vi "Pool.Destroy FIFO.vi"(8 "error in (no error)":errorcluster, 11 "Pool in":refnum<class "Pool.lvclass">) -> (0 "error out":errorcluster, 3 "Pool out":refnum<class "Pool.lvclass">)   [LabVIEW 2017, in "DSF.Engine.lvlib" / "Pool.lvclass"]
uses:
  Pool.lvclass
  Pool.lvclass/Pool.ctl
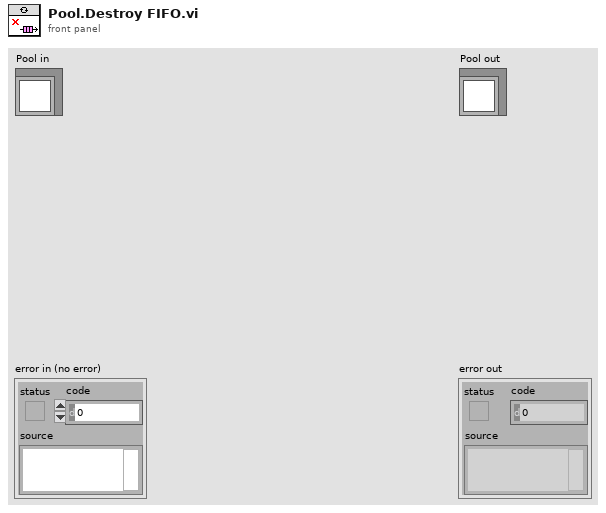
[diagram p1: front panel]
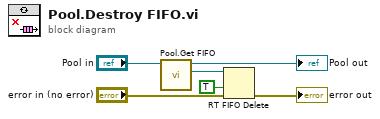
[diagram p0: block diagram]
diagram:
  n1 = call "Pool.Get FIFO.vi"("Pool in"="Pool in") -> ("FIFO"=w2:refnum<k33>, "Pool out"=→"Pool out":refnum<class "Pool.lvclass">)  [unwired: 9 in]
  n2 = RT FIFO Delete(0:w2, 2:TRUE ("force destroy? (F)"), 3:"error in (no error)") -> (11:→"error out":errorcluster)
